vi "cleanArrayRing.vi"(9 "index (row)":i32=2, 11 "array in":string[][](array[string])) -> (3 "Array out":cluster{"String":string, i32}[](array[cluster]))   [LabVIEW 2009]
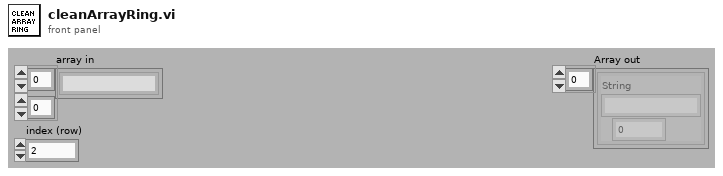
[diagram p1: front panel]
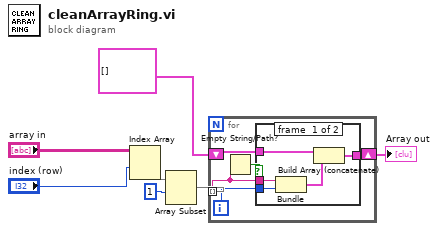
[diagram p0: block diagram]
diagram:
  n1 = Index Array(array="array in", index (row)="index (row)") -> (element=w6:string[])  [unwired: 1 in]
  n2 = Array Subset(array=w6, index=1) -> (w4:string[])  [unwired: 1 in]
  n3 = for {
    tunnel: w4 -> [w11] mode=indexing
    shift-right: [w9] -> w1
    shift-left: cluster{"String":string, i32}[] [] -> [w8]
    i -> [w12]
    n4 = Empty String/Path?(string/path=w11) -> (empty?=w10:bool)
    n5 = case shown="False" w10 {
      tunnel: w12 -> [w17 _]
      tunnel: w11 -> [w16 _]
      tunnel: [w14 w18] -> w9
      tunnel: w8 -> [w13 w18]
      frame #0 {
        n6 = Bundle("String"=w16, w17) -> (w15:cluster{"String":string, i32})  [unwired: 1 in]
        n7 = Build Array (concatenate)(w13, w15) -> (w14:cluster{"String":string, i32}[])
      }
      frame #1 {
      }
    }
  }
  "Array out" <- w1
